vi "Check_Traverse_move_Low.vi"(3 "Traverse Name":string, 5 "Exclude Array":T2[](array[typedef])=[{"Sizes"=[{"Max"=15000.0, "Min"=0.0}, {"Max"=1000.0, "Min"=-1000.0}, {"Max"=300.0, "Min"=0.0}], "Name"="Roughness Elements", "Exclude Type"=enum."Allow only vertical moves"}, {"Sizes"=[{"Max"=17000.0, "Min"=16000.0}, {"Max"=200.0, "Min"=-200.0}, {"Max"=-50.0, "Min"=-250.0}], "Name"="B204", "Exclude Type"=enum."Exclude completely"}] {"Sizes"."Min" format="%#.1f"; "Sizes"."Max" format="%#.1f"}, 6 "Probe Support":T1=[{"Max"=15001.0, "Min"=12000.0}, {"Max"=1000.0, "Min"=-1000.0}, {"Max"=700.0, "Min"=0.0}] {"Min" format="%#.1f"; "Max" format="%#.1f"}, 7 "Probe Volume":T1=[{"Max"=15.0, "Min"=-15.0}, {"Max"=250.0, "Min"=0.0}, {"Max"=15.0, "Min"=-15.0}] {"Min" format="%#.1f"; "Max" format="%#.1f"}, 8 "New Position":dbl[](array[numeric])=[0.0, 0.0, 0.0] format="%.2f", 9 "Current position":dbl[](array[numeric])=[0.0, 0.0, 0.0] format="%.2f") -> (0 "Error Comments":string, 2 "Position At Crash":dbl[](array[numeric]) format="%.2f")   [LabVIEW 2013]
uses:
  Box_size.ctl
  Exclude_cluster.ctl
  Exclusion_type.ctl
panel:
  out "Numeric":i32
  # "X                Y                   Z"
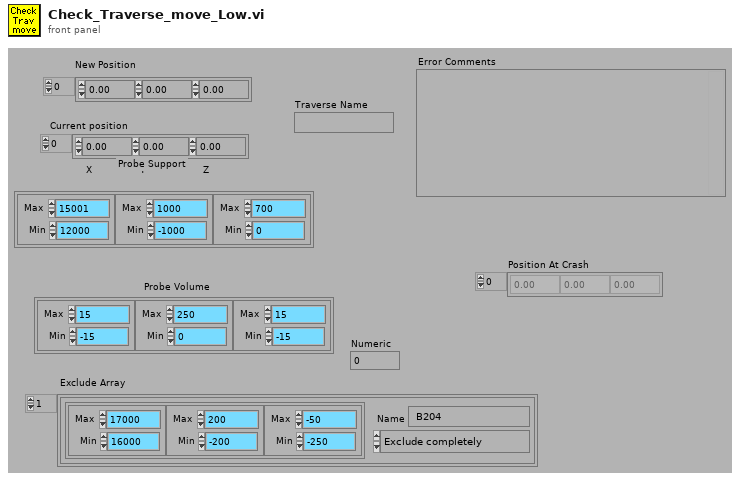
[diagram p1: front panel]
types:
  T1 = typedef "Box_size.ctl" = cluster{"Max":dbl, "Min":dbl}[]
  T2 = typedef "Exclude_cluster.ctl" = cluster{"Sizes":T1, "Name":string, "Exclude Type":T3}
  T3 = typedef "Exclusion_type.ctl" = enum16{"Exclude completely", "Allow only vertical moves"}
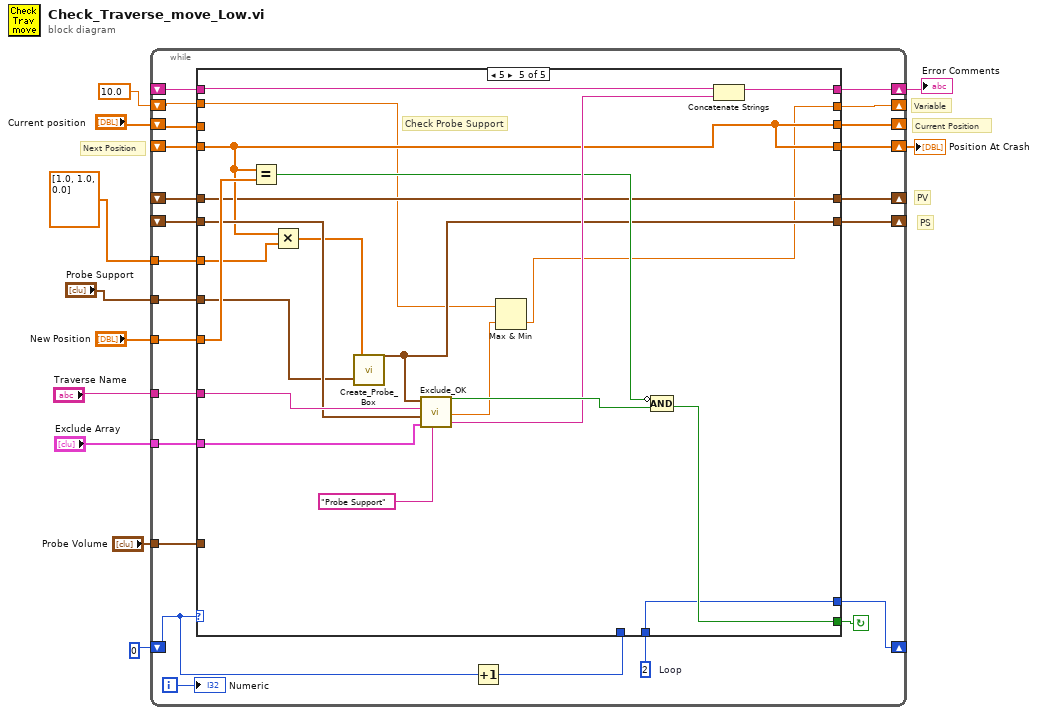
[diagram p0: block diagram]
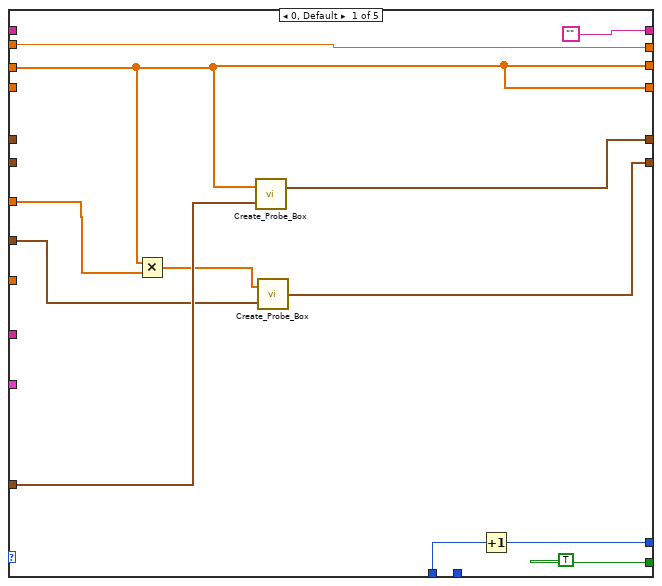
[diagram p2: hidden frame]
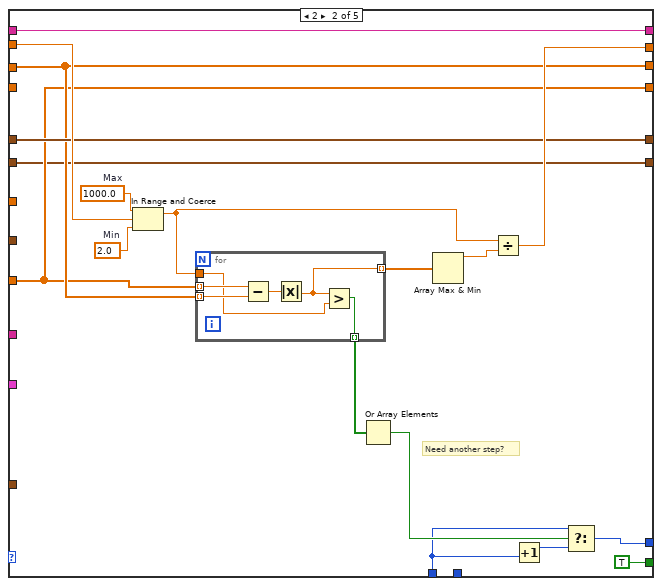
[diagram p3: hidden frame]
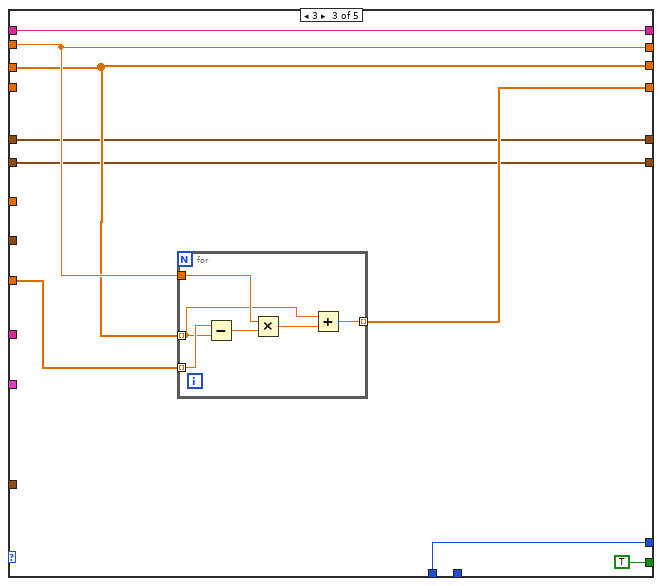
[diagram p4: hidden frame]
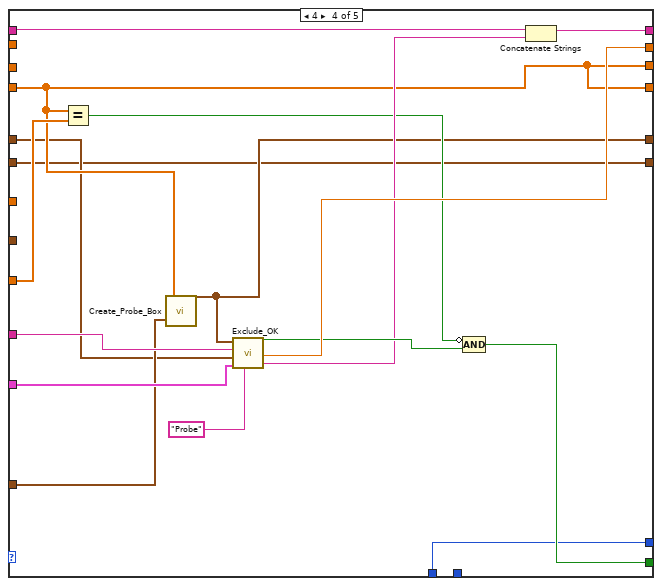
[diagram p5: hidden frame]
diagram:
  # "PS"
  # "PV"
  # "Current Position"
  # "Next Position"
  # "Variable"
  n1 = while {
    shift-left: _ -> [w16]
    shift-right: [w17] -> _
    tunnel: "Probe Volume" -> [w19]
    tunnel: "New Position" -> [w21]
    shift-left: _ -> [w23]
    shift-right: [w24] -> w7
    shift-left: 0 -> [w27]
    shift-right: [w26] -> _
    tunnel: "Traverse Name" -> [w28]
    tunnel: "Exclude Array" -> [w30]
    shift-left: 10.0 ("Separation Distance") -> [w34]
    shift-right: [w29] -> _
    shift-left: _ -> [w22]
    shift-right: [w32] -> w5
    shift-left: "Current position" -> [w35]
    shift-right: [w33] -> _
    shift-right: [w14] -> _
    shift-left: _ -> [w13]
    tunnel: "Probe Support" -> [w15]
    tunnel: dbl[] [1.0, 1.0, 0.0] ("Current position") -> [w12]
    i -> [w18]
    stop <- w31 continue-if-true
    w20 = 2  # Loop
    n2 = Increment(x=w27) -> (x+1=w25:i32)
    n3 = case shown="5" w27 {
      tunnel: w35 -> [w37 w51 w77 _ _]
      tunnel: w34 -> [w47 w65 w78 _ w106]
      tunnel: [w37 w51 w77 w94 w112] -> w33
      tunnel: [w37 w50 w76 w94 w112] -> w32
      tunnel: [TRUE ("Box Inside") TRUE ("Box Inside") TRUE ("Box Inside") w90 w116] -> w31
      tunnel: w19 -> [w45 _ _ w93 _]
      tunnel: w30 -> [_ _ _ w103 w124]
      tunnel: [w47 w57 w78 w102 w104] -> w29
      tunnel: w28 -> [_ _ _ w101 w123]
      tunnel: [w41 w55 w74 w89 w115] -> w26
      tunnel: w25 -> [w44 w53 w74 w89 _]
      tunnel: ["" w63 w80 w98 w120] -> w24
      tunnel: w23 -> [_ w63 w80 w99 w121]
      tunnel: w22 -> [_ _ _ w94 w112]
      tunnel: w21 -> [_ w50 w75 w96 w118]
      tunnel: w20 -> [_ _ _ _ w115]
      tunnel: [w42 w52 w73 w92 w108] -> w17
      tunnel: w16 -> [_ w52 w73 w91 w108]
      tunnel: w15 -> [w40 _ _ _ w113]
      tunnel: [w39 w48 w72 w88 w109] -> w14
      tunnel: w13 -> [_ w48 w72 w88 w114]
      tunnel: w12 -> [w38 _ _ _ w111]
      frame 0, Default {
        n4 = Multiply(x=w37, y=w38) -> (x*y=w36:dbl[])
        n5 = call "Create_Probe_Box.vi"("Probe Volume"=w45, "Probe Position"=w37) -> ("Current Probe Volume"=w42:cluster{"Max":dbl, "Min":dbl}[])
        n6 = call "Create_Probe_Box.vi"("Probe Volume"=w40, "Probe Position"=w36) -> ("Current Probe Volume"=w39:cluster{"Max":dbl, "Min":dbl}[])
        n7 = Increment(x=w44) -> (x+1=w41:i32)
      }
      frame 2 {
        w60 = 1000.0  # Max
        w61 = 2.0  # Min
        # "Need another step?"
        n8 = In Range and Coerce(upper limit=w60, x=w65, lower limit=w61) -> (coerced(x)=w49:dbl)  [unwired: 1 out]
        n9 = for {
          tunnel: w50 -> [w71] mode=indexing
          tunnel: w51 -> [w70] mode=indexing
          tunnel: w49 -> [w69]
          tunnel: [w67] -> w62 mode=indexing
          tunnel: [w66] -> w59 mode=indexing
          n10 = Subtract(x=w71, y=w70) -> (x-y=w68:dbl)
          n11 = Absolute Value(x=w68) -> (abs(x)=w66:dbl)
          n12 = Greater?(x=w66, y=w69) -> (0:w67:bool)
        }
        n13 = Or Array Elements(Boolean array=w62) -> (logical OR=w56:bool)
        n14 = Array Max & Min(array=w59) -> (max value=w58:dbl)  [unwired: 3 out]
        n15 = Divide(x=w49, y=w58) -> (x/y=w57:dbl)
        n16 = Increment(x=w53) -> (x+1=w54:i32)
        n17 = Select(t=w53, s=w56, f=w54) -> (s? t:f=w55:i32)
      }
      frame 3 {
        n18 = for {
          tunnel: w75 -> [w86] mode=indexing
          tunnel: w77 -> [w82] mode=indexing
          tunnel: w78 -> [w84]
          tunnel: [w81] -> w76 mode=indexing
          n19 = Subtract(x=w86, y=w82) -> (x-y=w85:dbl)
          n20 = Multiply(x=w84, y=w85) -> (x*y=w83:dbl)
          n21 = Add(x=w82, y=w83) -> (x+y=w81:dbl)
        }
      }
      frame 4 {
        n22 = Equal?(x=w94, y=w96) -> (x = y?=w95:bool)
        n23 = call "Create_Probe_Box.vi"("Probe Volume"=w93, "Probe Position"=w94) -> ("Current Probe Volume"=w92:cluster{"Max":dbl, "Min":dbl}[])
        n24 = call "Exclude_OK.vi"("Probe Volume"=w92, "Traverse Name"=w101, "Previous Probe Volume"=w91, "Exclude Array"=w103, "Volume Name"="Probe") -> ("Probe OK?"=w100:bool, "Separation Distance"=w102:dbl, "Error Comments"=w97:string)
        n25 = Compound Arithmetic op=AND(invert w95, w100) -> (w90:bool)
        n26 = Concatenate Strings(w99, w97) -> (w98:string)
      }
      frame 5 {
        # "Check Probe Support"
        n27 = Equal?(x=w112, y=w118) -> (x = y?=w117:bool)
        n28 = Multiply(x=w112, y=w111) -> (x*y=w110:dbl[])
        n29 = call "Create_Probe_Box.vi"("Probe Volume"=w113, "Probe Position"=w110) -> ("Current Probe Volume"=w109:cluster{"Max":dbl, "Min":dbl}[])
        n30 = call "Exclude_OK.vi"("Probe Volume"=w109, "Traverse Name"=w123, "Previous Probe Volume"=w114, "Exclude Array"=w124, "Volume Name"="Probe Support") -> ("Probe OK?"=w122:bool, "Separation Distance"=w105:dbl, "Error Comments"=w119:string)
        n31 = Max & Min(x=w106, y=w105) -> (min(x,y)=w104:dbl)  [unwired: 1 out]
        n32 = Compound Arithmetic op=AND(invert w117, w122) -> (w116:bool)
        n33 = Concatenate Strings(w121, w119) -> (w120:string)
      }
    }
    "Numeric" <- w18
  }
  "Error Comments" <- w7
  "Position At Crash" <- w5
